vi "NI-Switch Specific Logic.vi"(8 "error in":errorcluster, 10 "session factory in":refnum<class "Session Factory.lvclass">, 11 "measurement configuration":T1={"relay name"="", "channel"="", "relay action"=21} {"relay action" items=["Open Relay"=20, "Close Relay"=21]}) -> (0 "error out":errorcluster, 3 "measurement results":T3={"initial relay position"=10, "final relay position"=10} {"final relay position" items=["Open"=10, "Closed"=11]; "initial relay position" items=["Open"=10, "Closed"=11]})   [LabVIEW 2021, in "NI-Switch Control Relay.lvlib"]
uses:
  NI-Switch Control Relay.lvlib
  Source/Sessions/niSwitch/Session Factory/Session Factory.lvclass
  Measurement Results.ctl
  <instrlib>/niSwitch/niSwitch.llb/niSwitch Relay Position.ctl
  Measurement Configuration.ctl
  <instrlib>/niSwitch/niSwitch.llb/niSwitch Relay Action.ctl
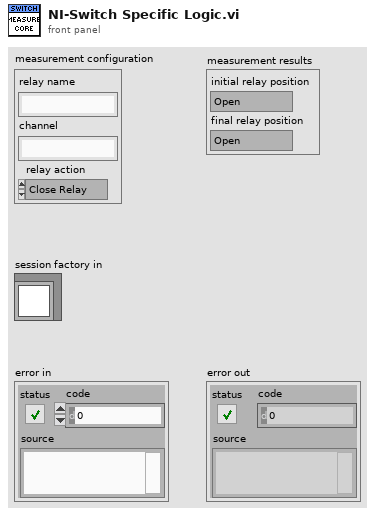
[diagram p1: front panel]
types:
  T1 = typedef "NI-Switch Control Relay.lvlib/Measurement Configuration.ctl" = cluster{"relay name":string, "channel":string, "relay action":T2}
  T2 = typedef "niSwitch Relay Action.ctl" = i32
  T3 = typedef "NI-Switch Control Relay.lvlib/Measurement Results.ctl" = cluster{"initial relay position":T4, "final relay position":T4}
  T4 = typedef "niSwitch Relay Position.ctl" = i32
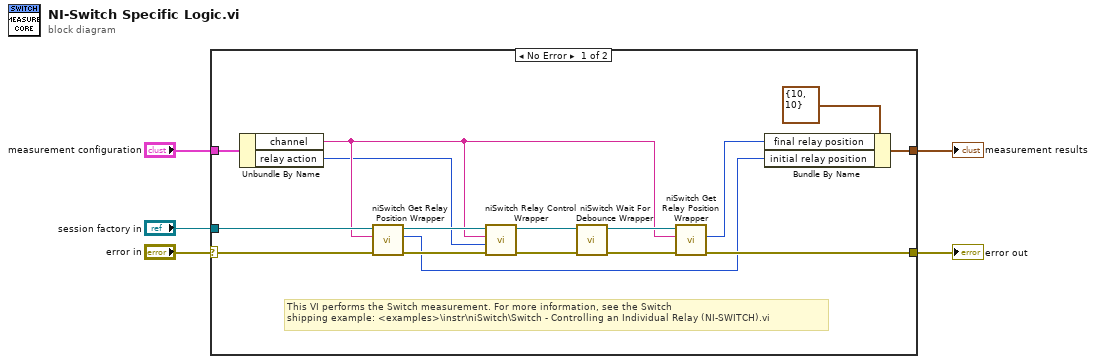
[diagram p0: block diagram]
diagram:
  n1 = case shown="No Error" "error in" {
    selector: "error in" -> [w17 w22]
    tunnel: "session factory in" -> [w18 _]
    tunnel: [w13 w22] -> w1
    tunnel: "measurement configuration" -> [w12 _]
    tunnel: [w7 _] -> w2
    frame No Error {
      # "This VI performs the Switch measurement. For more information, see the Switch\nshipping example: <examples>\\instr\\niSwitch\\Switch - Controlling an Individual Relay (NI-SWITCH).vi"
      n2 = Unbundle By Name(w12) -> ("channel"=w11:string, "relay action"=w10:T2)
      n3 = call "niSwitch Get Relay Position Wrapper.vi"("error in"=w17, "relay name"=w11, "session factory in"=w18) -> ("error out"=w16:errorcluster, "position"=w8:T4, "session factory out"=w21:refnum<class "Session Factory.lvclass">)  [unwired: 6 in]
      n4 = call "niSwitch Relay Control Wrapper.vi"("error in"=w16, "relay action (Close Relay)"=w10, "relay names"=w11, "session factory in"=w21) -> ("error out"=w15:errorcluster, "session factory out"=w20:refnum<class "Session Factory.lvclass">)  [unwired: 6 in]
      n5 = call "niSwitch Wait For Debounce Wrapper.vi"("error in"=w15, "session factory in"=w20) -> ("error out"=w14:errorcluster, "session factory out"=w19:refnum<class "Session Factory.lvclass">)  [unwired: 8 in]
      n6 = call "niSwitch Get Relay Position Wrapper.vi"("error in"=w14, "relay name"=w11, "session factory in"=w19) -> ("error out"=w13:errorcluster, "position"=w9:T4)  [unwired: 6 in, 1 out]
      n7 = Bundle By Name(cluster=T3 {"initial relay position"=10, "final relay position"=10} ("measurement results"), "final relay position"=w9, "initial relay position"=w8) -> (w7:T3)
    }
    frame Error {
    }
  }
  "error out" <- w1
  "measurement results" <- w2
